vi "PrepareHWI.vi"(8 "error in (no error)":errorcluster, 9 "Master Device in":refnum<class "Master Device.lvclass">, 10 "Current Variables":T1[](array[typedef]), 11 "SRS_DS345 in":refnum<class "SRS_DS345.lvclass">) -> (0 "error out":errorcluster, 2 "Master Device out":refnum<class "Master Device.lvclass">, 3 "SRS_DS345 out":refnum<class "SRS_DS345.lvclass">)   [LabVIEW 2013, in "SRS_DS345.lvclass"]
doc: "Prepare HWI will parse string table values to generate a hardware image for each device. Both variables and user functions can be pre-registered! This makes setting variables optional."
uses:
  SRS_DS345.lvclass
  TypeDefs/Active procedure variables.ctl
  Master Device/Master Device.lvclass
  ColumnVIs/MenuCol/MenuCol.lvclass
  SRS_DS345.lvclass/SRS_DS345.ctl
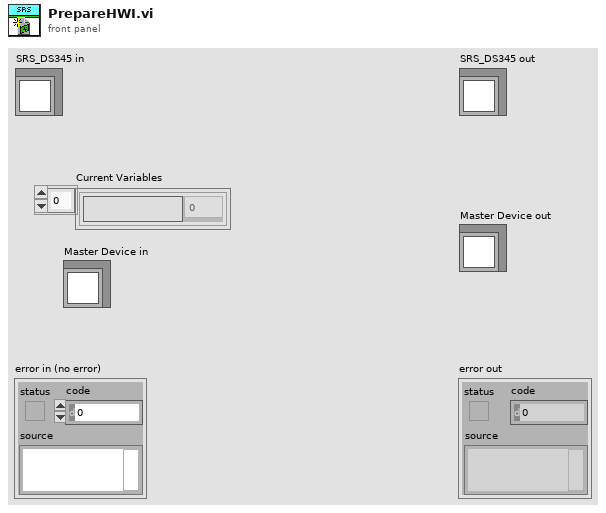
[diagram p1: front panel]
types:
  T1 = typedef "Active procedure variables.ctl" = cluster{"Procedure variable":string, "Value":dbl}
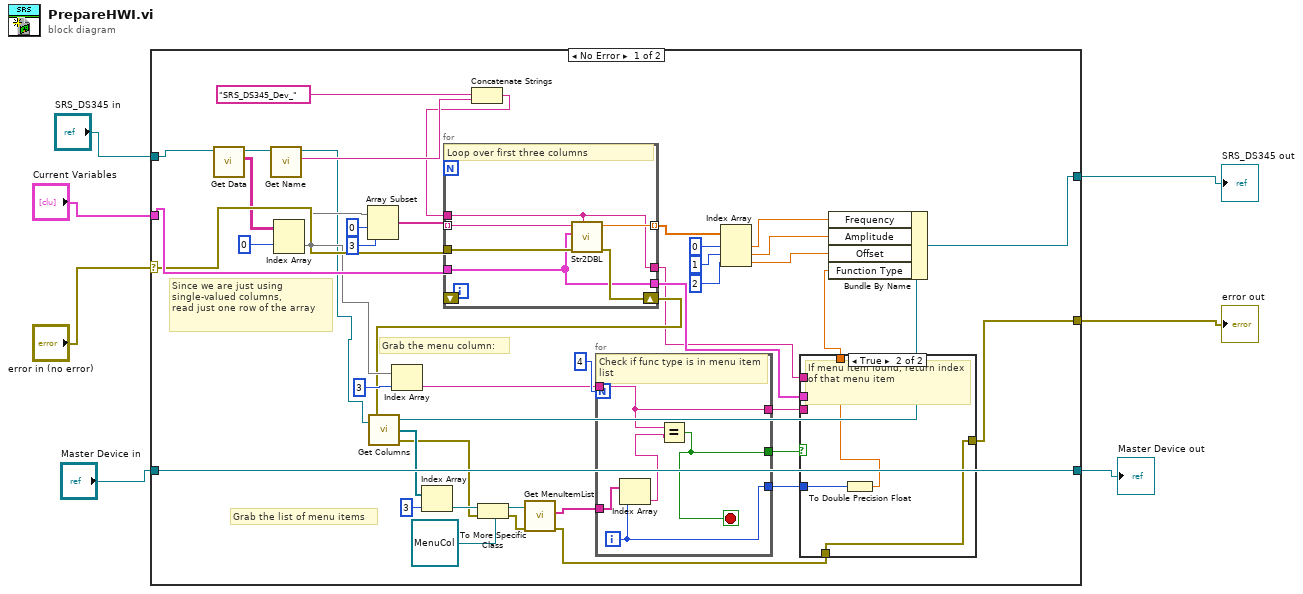
[diagram p0: block diagram]
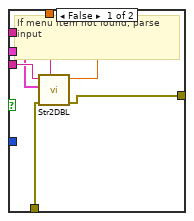
[diagram p2: hidden frame]
diagram:
  n1 = case shown="No Error" "error in (no error)" {
    selector: "error in (no error)" -> [w44 w74]
    tunnel: [w12 w74] -> w1
    tunnel: "Master Device in" -> [w51 w73]
    tunnel: [w51 w73] -> w5
    tunnel: "SRS_DS345 in" -> [w50 w72]
    tunnel: [w37 w72] -> w6
    tunnel: "Current Variables" -> [w45 _]
    frame No Error {
      # "Grab the list of menu items"
      # "Grab the menu column:"
      # "Since we are just using single-valued columns, \nread just one row of the array"
      n2 = call-dynamic "Get Data.vi"("Device in"=w50) -> ("Table Indicator"=w43:string[][], "Device out"=w49:refnum<class "SRS_DS345.lvclass">)  [unwired: 7 in, 1 out]
      n3 = call-dynamic "Get Name.vi"("Device in"=w49) -> ("Name"=w48:string, "Device out"=w28:refnum<class "SRS_DS345.lvclass">)  [unwired: 8 in, 1 out]
      n4 = Index Array(array=w43, index (row)=0) -> (element=w30:string[])  [unwired: 1 in]
      n5 = Array Subset(array=w30, index=0, length=3) -> (w31:string[])
      n6 = Index Array(array=w30, index=3) -> (element=w19:string)
      n7 = Concatenate Strings("SRS_DS345_Dev_", w48) -> (w46:string)
      n8 = for {
        tunnel: w46 -> [w66]
        tunnel: w45 -> [w67]
        tunnel: w44 -> [w71]
        tunnel: w31 -> [w70] mode=indexing
        tunnel: [w69] -> w41 mode=indexing
        shift-right: [w68] -> w22
        shift-left: _ -> [_]
        tunnel: [w67] -> w14
        tunnel: [w66] -> w13
        # "Loop over first three columns"
        n9 = call "Str2DBL.vi"("Error Locator"=w66, "error in (no error)"=w71, "Current Variable settings"=w67, "formula"=w70) -> ("error out"=w68:errorcluster, "y value"=w69:dbl)  [unwired: 4 in]
      }
      n10 = call-dynamic "Get Columns.vi"("Device in"=w28, "error in (no error)"=w22) -> ("Device out"=w27:refnum<class "SRS_DS345.lvclass">, "Columns"=w26:refnum<class "Column.lvclass">[], "error out"=w21:errorcluster)
      n11 = Index Array(array=w26, index=3) -> (element=w23:refnum<class "Column.lvclass">)
      n12 = To More Specific Class(target class=refnum<class "MenuCol.lvclass"> refnum ("MenuCol.lvclass"), reference=w23, error in=w21) -> (specific class reference=w11:refnum<class "MenuCol.lvclass">, error out=w10:errorcluster)
      n13 = call-dynamic "Get MenuItemList.vi"("error in (no error)"=w10, "MenuCol in"=w11) -> ("error out"=w8:errorcluster, "MenuItemList"=w9:string[])  [unwired: 7 in, 1 out]
      n14 = for {
        N: 4 -> [_]
        tunnel: w19 -> [w62]
        tunnel: w9 -> [w65]
        tunnel: [w64] -> w17
        tunnel: [w61] -> w18
        tunnel: [w62] -> w15
        i -> [w64]
        stop <- w61 stop-if-true
        # "Check if func type is in menu item list"
        n15 = Index Array(array=w65, index=w64) -> (element=w63:string)
        n16 = Equal?(x=w62, y=w63) -> (x = y?=w61:bool)
      }
      n17 = Index Array(array=w41, index #1=0 ("index"), index #2=1 ("index"), index #3=2 ("index")) -> (element #1=w36:dbl, element #2=w35:dbl, element #3=w34:dbl)
      n18 = case shown="True" w18 {
        tunnel: w17 -> [_ w58]
        tunnel: [w52 w59] -> w16
        tunnel: w15 -> [w57 _]
        tunnel: w14 -> [w56 _]
        tunnel: w13 -> [w55 _]
        tunnel: w8 -> [w54 w60]
        tunnel: [w53 w60] -> w12
        frame False {
          # "If menu item not found, parse input"
          n19 = call "Str2DBL.vi"("Error Locator"=w55, "error in (no error)"=w54, "Current Variable settings"=w56, "formula"=w57) -> ("error out"=w53:errorcluster, "y value"=w52:dbl)  [unwired: 4 in]
        }
        frame True {
          # "If menu item found, return index of that menu item"
          n20 = To Double Precision Float(number=w58) -> (double precision float=w59:dbl)
        }
      }
      n21 = Bundle By Name(cluster=w27, "Frequency"=w36, "Amplitude"=w35, "Offset"=w34, "Function Type"=w16) -> (w37:refnum<class "SRS_DS345.lvclass">)
    }
    frame Error {
    }
  }
  "error out" <- w1
  "SRS_DS345 out" <- w6
  "Master Device out" <- w5
